vi "Example Loopback.vi"() -> ()   [LabVIEW 2010]
uses:
  C:/tf/play/labview/Tinkerforge.dll
  Tinkerforge.dll
panel:
  out "message":string
  in  "stop":bool
  in  "uid":string="amb"
  in  "port":i32=4223
  in  "host":string="localhost"
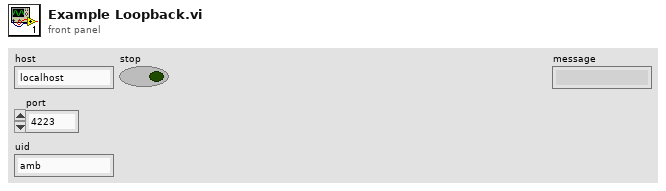
[diagram p1: front panel]
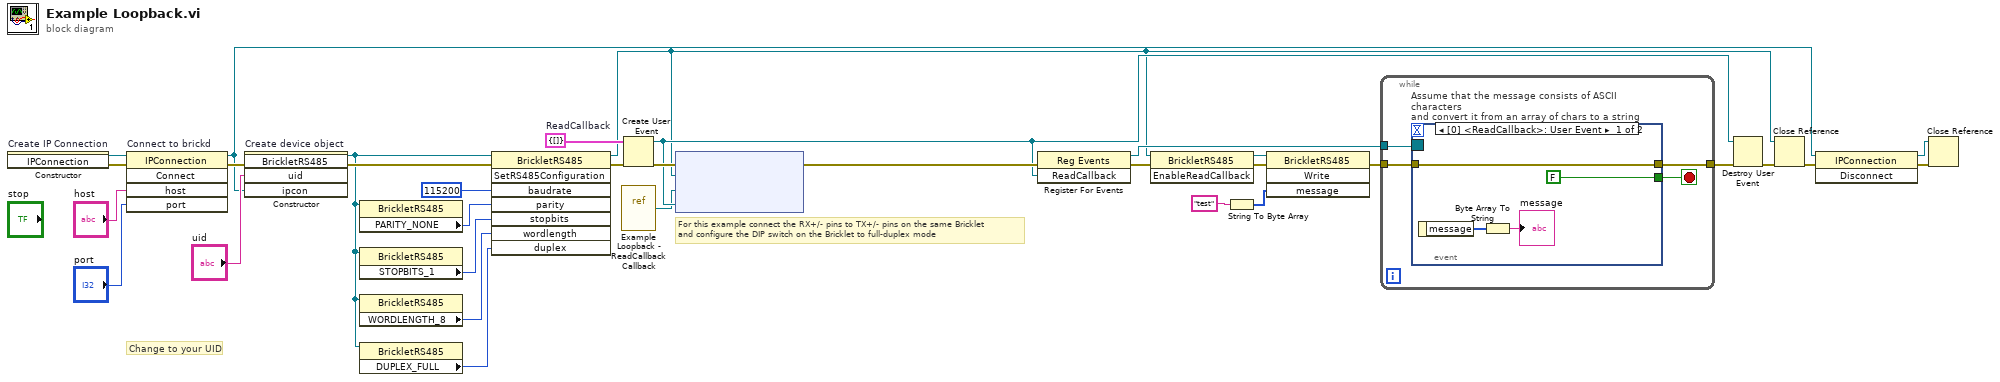
[diagram p0: block diagram]
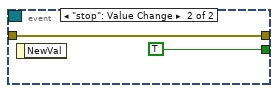
[diagram p2: hidden frame]
diagram:
  w17 = cluster{"message":u16[]} {"message"=[]}  # ReadCallback
  # "For this example connect the RX+/- pins to TX+/- pins on the same Bricklet\nand configure the DIP switch on the Bricklet to full-duplex mode"
  # "Change to your UID"
  n1 = constructor on="Create IP Connection" class="IPConnection"() -> (reference out=w33:refnum<k24>, error out=w18:errorcluster)  [unwired: 3 in, 1 out]
  n2 = invoke on="Connect to brickd" class="IPConnection" method="Connect"(reference=w33, error in=w18, "host"="host", "port"="port") -> (reference out=w26:refnum<k24>, error out=w29:errorcluster)  [unwired: 1 in, 3 out]
  n3 = constructor on="Create device object" class="BrickletRS485"(error in=w29, "uid"="uid", "ipcon"=w26) -> (reference out=w1:refnum<k24>, error out=w5:errorcluster)  [unwired: 2 in, 3 out]
  n4 = property class="BrickletRS485"(reference=w1) -> ("PARITY_NONE"=w2:u8)  [unwired: 1 in, 2 out]
  n5 = property class="BrickletRS485"(reference=w1) -> ("STOPBITS_1"=w3:u8)  [unwired: 1 in, 2 out]
  n6 = property class="BrickletRS485"(reference=w1) -> ("WORDLENGTH_8"=w6:u8)  [unwired: 1 in, 2 out]
  n7 = property class="BrickletRS485"(reference=w1) -> ("DUPLEX_FULL"=w7:u8)  [unwired: 1 in, 2 out]
  n8 = invoke class="BrickletRS485" method="SetRS485Configuration"(reference=w1, error in=w5, "baudrate"=i64 115200, "parity"=w2, "stopbits"=w3, "wordlength"=w6, "duplex"=w7) -> (reference out=w8:refnum<k24>, error out=w9:errorcluster)  [unwired: 1 in, 6 out]
  n9 = vi-ref "Example Loopback - ReadCallback Callback.vi"() -> ("vi reference"=w10:refnum<vi>)
  n10 = Create User Event(user event datatype=w17, error in=w9) -> (user event=w20:refnum<user-event>, error out=w24:errorcluster)
  n11 = node ("Register Event Callback")(w24, w8, w10, w20) -> (w23:errorcluster)  [unwired: 1 in, 1 out]
  n12 = register-events(error in=w23, w20) -> (reference out=w22:refnum<event-registration>, error out=w16:errorcluster)  [unwired: 1 in]
  n13 = invoke class="BrickletRS485" method="EnableReadCallback"(reference=w8, error in=w16) -> (reference out=w13:refnum<k24>, error out=w15:errorcluster)  [unwired: 1 in, 1 out]
  n14 = String To Byte Array(string="test") -> (unsigned byte array=w11:u8[])
  n15 = invoke class="BrickletRS485" method="Write"(reference=w13, error in=w15, "message"=w11) -> (error out=w14:errorcluster)  [unwired: 1 in, 3 out]
  n16 = while {
    tunnel: w22 -> [w37]
    tunnel: [w36] -> w21
    tunnel: w14 -> [w35]
    stop <- w34 stop-if-true
    n17 = event "Assume that the message consists of ASCII characters\nand convert it from an array of chars to a string" shown="[0] <ReadCallback>: User Event" {
      selector: w37 -> [_ _]
      dyn-events: _ -> [_ _]
      timeout: _ -> [_ _]
      tunnel: [w41 w42] -> w36
      tunnel: w35 -> [w41 w42]
      tunnel: [FALSE TRUE] -> w34
      event User Event {
        n18 = event-data() -> ("message"=w38:u16[])  [unwired: 1 in]
        n19 = Byte Array To String(unsigned byte array=w38) -> (string=→"message":string)
      }
      event "stop": Value Change {
        n20 = event-data() -> ()  [unwired: 1 in, 1 out]
      }
    }
  }
  n21 = Destroy User Event(user event=w20, error in=w21) -> (error out=w19:errorcluster)
  n22 = Close Reference(reference=w8, error in (no error)=w19) -> (error out=w28:errorcluster)
  n23 = invoke class="IPConnection" method="Disconnect"(reference=w26, error in=w28) -> (reference out=w25:refnum<k24>, error out=w27:errorcluster)  [unwired: 1 in, 1 out]
  n24 = Close Reference(reference=w25, error in (no error)=w27) -> ()  [unwired: 1 out]
